vi "UpdateValues.vi"(8 "error in (no error)":errorcluster, 10 "Delta":i32, 11 "Panel_UI in":refnum<class "Panel_UI.lvclass">) -> (0 "error out":errorcluster, 3 "Panel_UI out":refnum<class "Panel_UI.lvclass">)   [LabVIEW 2015, in "Panel_UI.lvclass"]
uses:
  Panel_UI.lvclass
  Panel_UI.lvclass/Panel_UI.ctl
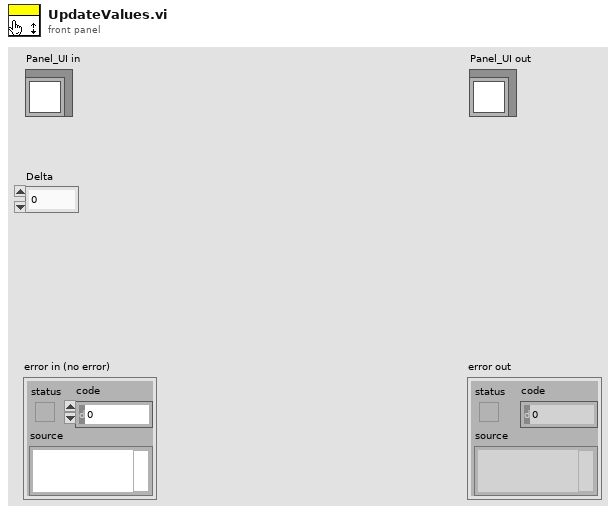
[diagram p1: front panel]
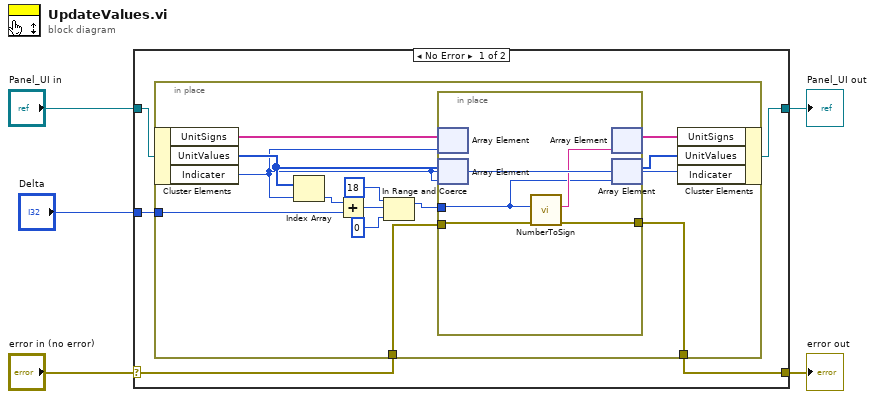
[diagram p0: block diagram]
diagram:
  n1 = case shown="No Error" "error in (no error)" {
    selector: "error in (no error)" -> [w9 w29]
    tunnel: [w8 w29] -> w4
    tunnel: [w6 w28] -> w2
    tunnel: "Panel_UI in" -> [w7 w28]
    tunnel: "Delta" -> [w10 _]
    frame No Error {
      n2 = in-place {
        in-place-border: w10 -> [w15]
        in-place-border: w9 -> [w22]
        in-place-border: [w21] -> w8
        n3 = in-place-cluster #1(w7) -> ("UnitSigns"=w20:string[], "UnitValues"=w19:i32[], "Indicater"=w16:i32)
        n4 = Index Array(array=w19, index=w16) -> (element=w23:i32)
        n5 = Add(x=w23, y=w15) -> (x+y=w14:i32)
        n6 = In Range and Coerce(upper limit=18, x=w14, lower limit=0) -> (coerced(x)=w11:i32)  [unwired: 1 out]
        n7 = in-place {
          in-place-border: w11 -> [w24]
          in-place-border: w22 -> [w27]
          in-place-border: [w25] -> w21
          n8 = in-place-array #2(w20, w16) -> ()  [unwired: 1 out]
          n9 = in-place-array #3(w19, w16) -> ()  [unwired: 1 out]
          n10 = call "NumberToSign.vi"("error in (no error)"=w27, "Number"=w24) -> ("error out"=w25:errorcluster, "Display"=w26:string)  [unwired: 8 in]
          n11 = in-place-array #2(w26) -> (w18:string[])  [unwired: 1 out]
          n12 = in-place-array #3(w24) -> (w17:i32[])  [unwired: 1 out]
        }
        n13 = in-place-cluster #1("UnitSigns"=w18, "UnitValues"=w17, "Indicater"=w16) -> (w6:refnum<class "Panel_UI.lvclass">)
      }
    }
    frame Error {
    }
  }
  "error out" <- w4
  "Panel_UI out" <- w2
